vi "DataViewerMain_20190214.vi"() -> ()   [LabVIEW 2018]
uses:
  DataViewerStatesEnum.ctl
  HDF5/HDF5_NoiseInfoClust.ctl
  HDF5/TC_Data_Structure.ctl
  HDF5/HDF5_TC_Errors.ctl
  HDF5/AI_alarm_data_cluster.ctl
  <vilib>/addons/h5labview2/file/H5Fmode.ctl
  ItemsInFile_Clust.ctl
  <vilib>/addons/h5labview2/file/H5F.lvlib
  <vilib>/addons/h5labview2/group/H5G.lvlib
panel:
  in  "File Selection":string[](tree)
  out "Item Value":dbl[][](graph) caption="Beac_MaxValue"
  in  "1 Hz?":bool
  out "TimeStamp":dbl[](array[numeric])
  out "TimeString (High)":string[](array[string])
  in  "ReLoad Data":bool
  in  "Index#":cluster{dbl, dbl}(slide)={0.0, 2963.282178217822} scale=0.0..23219.0
  out "Current Time":timestamp
  in  "Exit":bool
  in  "Load Data":bool
  in  "Start Crawl":bool
  out "TimeString (Low)":string[](array[string])
  in  "Channel Selection":string[](tree)
  in  "path":path=path "C:/ConnexData"
  # "Ver 2019_05_28"
  # "Select a folder\n(Not an individual file)"
  # "Click Start Folder Crawl"
  # "Select a group, then \ndata set, then one or more\ndata files."
  # "Select whether the data is\non a 1 second or\n1 minute time scale"
  # "Click Load Selected Data"
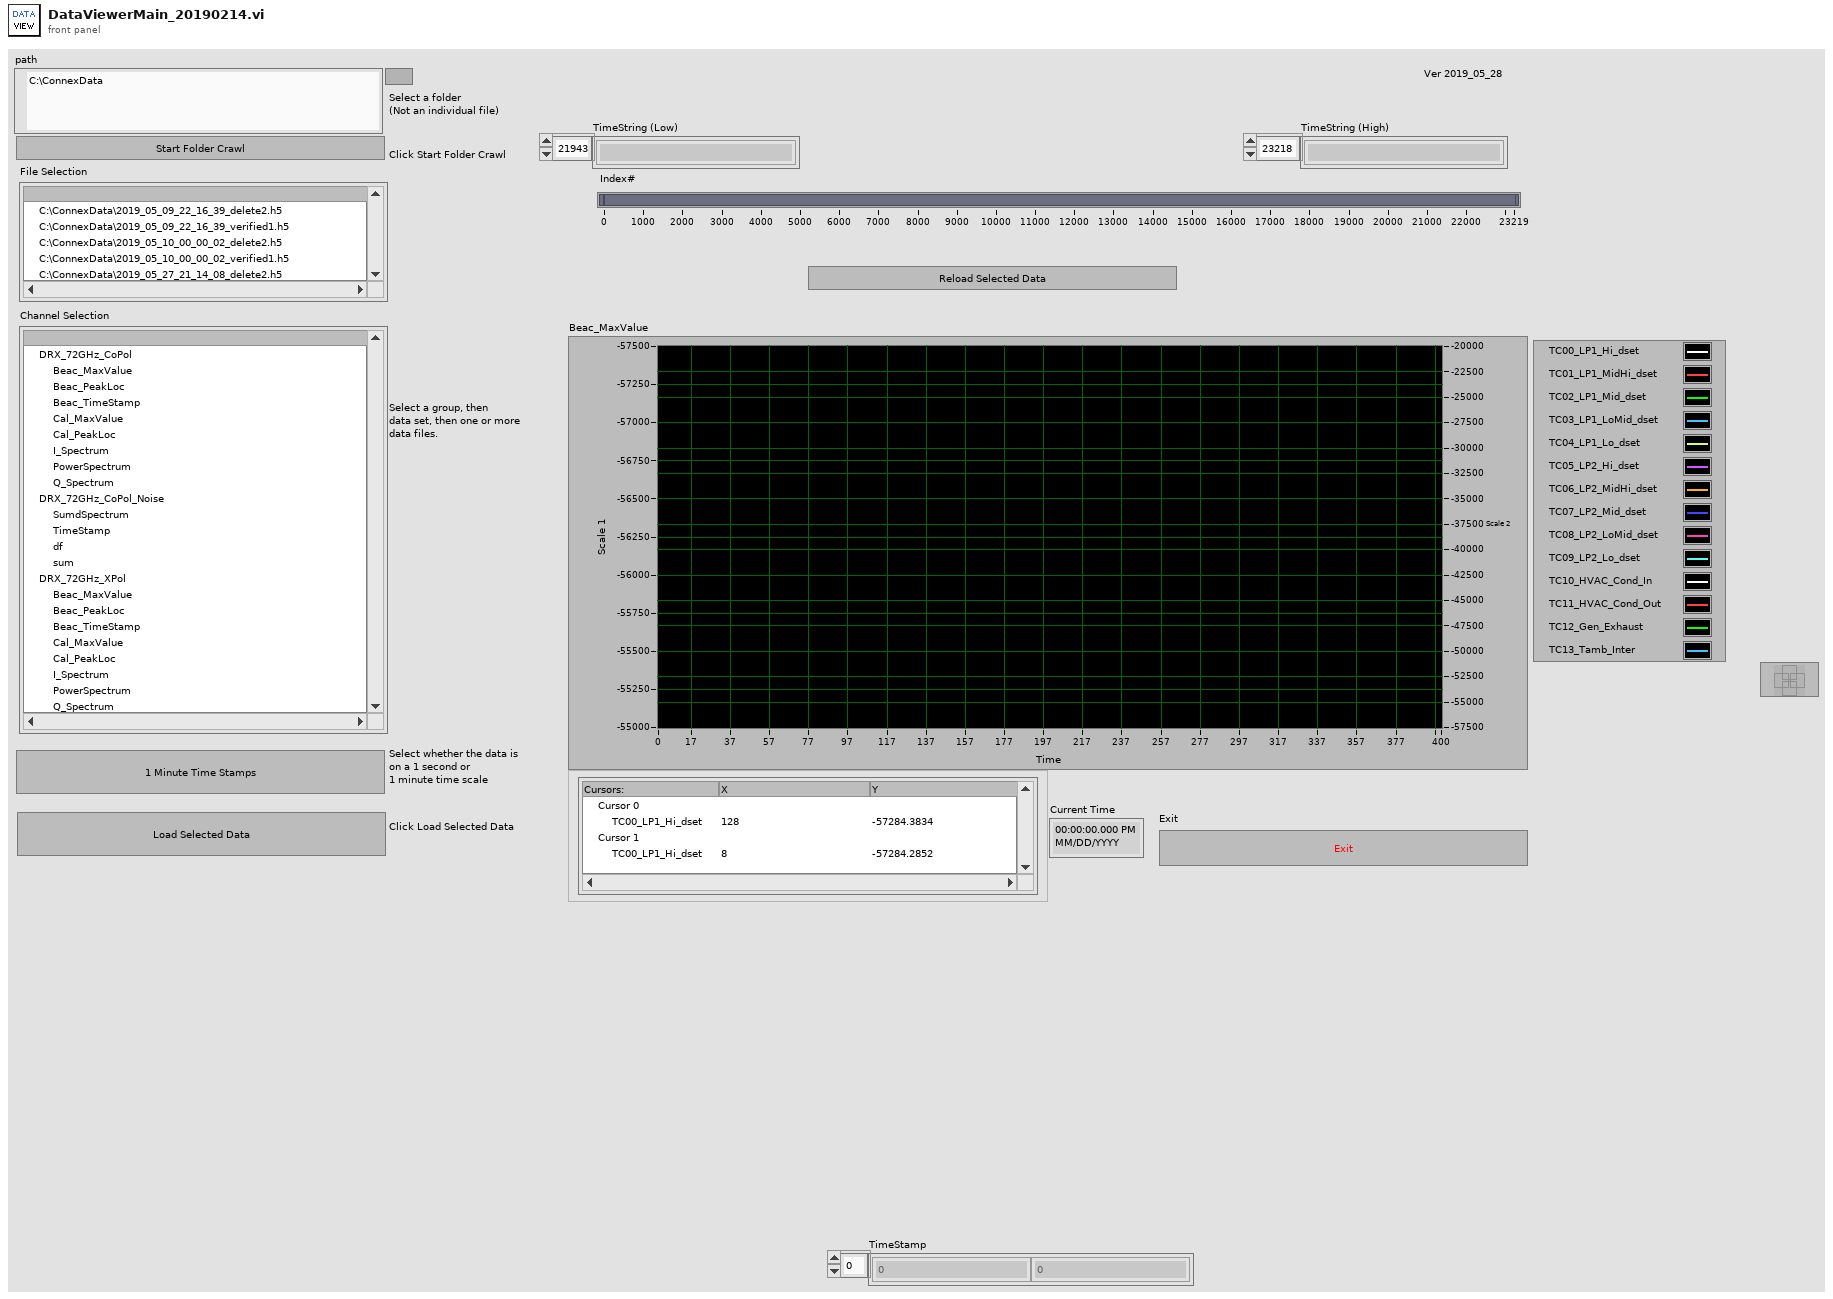
[diagram p1: front panel]
types:
  T1 = typedef "DataViewerStatesEnum.ctl" = enum16{"Idle", "Init", "CrawlFolders", "ListAllObjects", "PopulateTree", "LoadItemValues", "LoadBeacCalZoom", "LoadAlarms", "TimeShift", "Exit"}
  T2 = typedef "AI_alarm_data_cluster.ctl" = cluster{"current time":dbl, "date/time string":string, "AI 0":dbl, "AI 1":dbl, "AI 2":dbl, "AI 3":dbl, "AI 4":dbl, "AI 5":dbl, "AI 6":dbl, "AI 7":dbl, "AI 16":dbl, "AI 17":dbl, "AI 18":dbl, "AI 19":dbl, "AI 20":dbl, "AI 21":dbl, "AI 22":dbl, "AI 23":dbl}
  T3 = typedef "HDF5_TC_Errors.ctl" = cluster{"current time":dbl, "date/time string":string, "TC 0":dbl, "TC 1":dbl, "TC 2":dbl, "TC 3":dbl, "TC 4":dbl, "TC 5":dbl, "TC 6":dbl, "TC 7":dbl, "TC 8":dbl, "TC 9":dbl, "TC 10":dbl, "TC 11":dbl, "TC 12":dbl, "TC 13":dbl, "TC 14":dbl, "TC 15":dbl, "TC 16":dbl, "TC 17":dbl, "TC 18":dbl, "TC 19":dbl, "TC 20":dbl}
  T4 = typedef "TC_Data_Structure.ctl" = cluster{"TimeStamp":dbl, "TimeString":string, "TC0_LP1_Hi":dbl, "TC1_LP1_MidHi":dbl, "TC2_LP1_Mid":dbl, "TC3_LP1_LoMid":dbl, "TC4_LP1_Lo":dbl, "TC5_LP2_Hi":dbl, "TC6_LP2_MidHi":dbl, "TC7_LP2_Mid":dbl, "TC8_LP2_LoMid":dbl, "TC9_LP2_Lo":dbl, "TC10_HVAC_Cond_In":dbl, "TC11_HVAC_Cond_Out":dbl, "TC12_Gen_Exhaust":dbl, "TC13_Unused":dbl, "TC14_Unused":dbl, "TC15_Unused":dbl, "TC16_Unused":dbl, "TC17_Unused":dbl, "TC18_Unused":dbl, "TC19_Unused":dbl, "TC20_Unused":dbl, "TC21_Unused":dbl, "TC22_Unused":dbl, "TC23_Unused":dbl, "TC24_Unused":dbl, "TC25_Unused":dbl, "TC26_Unused":dbl, "TC27_Unused":dbl, "TC28_Unused":dbl, "TC29_Unused":dbl, "TC30_Unused":dbl, "TC31_Unused":dbl}
  T5 = typedef "HDF5_NoiseInfoClust.ctl" = cluster{"Timestring":string, "Timestamp":dbl, "df":dbl, "Sum":dbl}
  T6 = typedef "ItemsInFile_Clust.ctl" = cluster{"Group":string[], "Channel":string[][], "FilePath":string[]}
  T7 = typedef "H5F.lvlib/H5Fmode.ctl" = enum16{"read-only", "read-write", "overwrite", "create new", "open or create"}
  T8 = typedef "hid_t.ctl" = i32
  T9 = typedef "h5o_type.ctl" = enum8{"Group", "Dataset", "Named type"}
  T10 = cluster{"Left Cell String":string, "Child Text":string[], "Child Tag":string, "Item Indent":i32, "Child Only?":bool, "Glyph Index":i32}[]
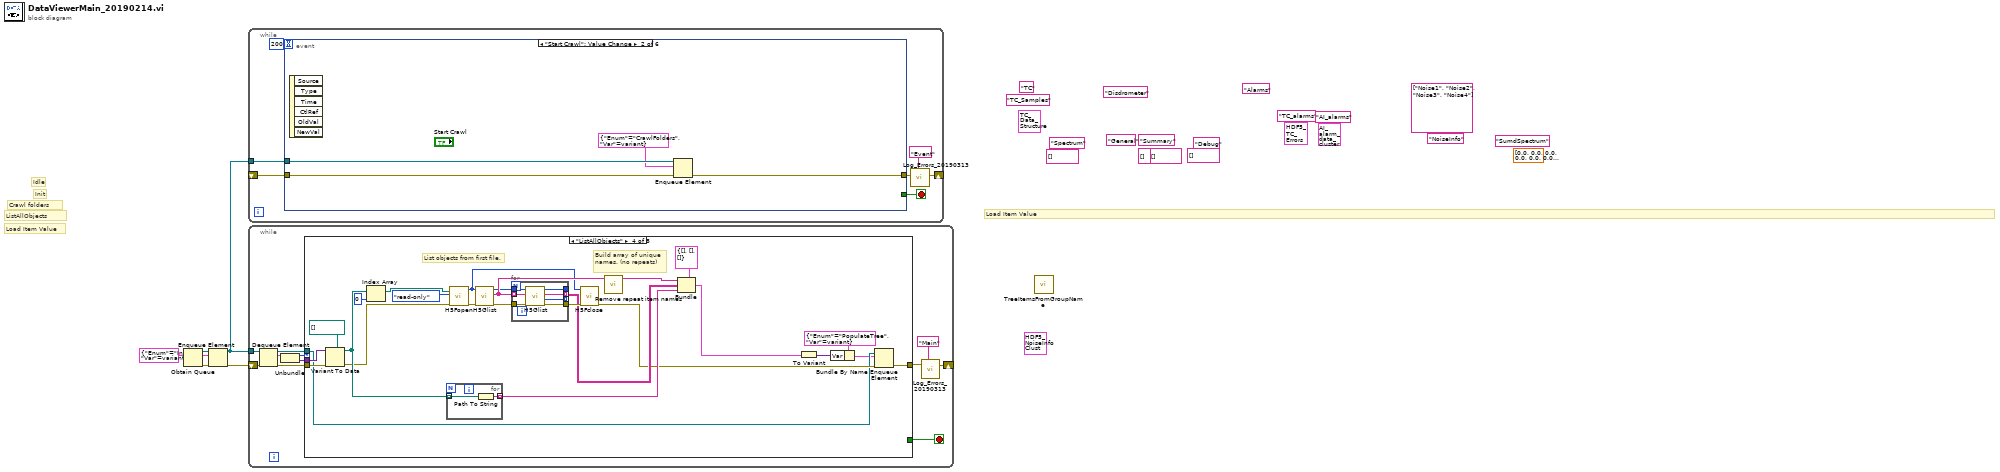
[diagram p0: block diagram]
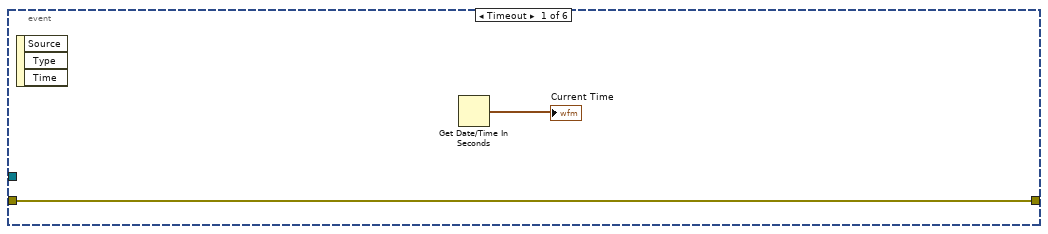
[diagram p2: hidden frame]
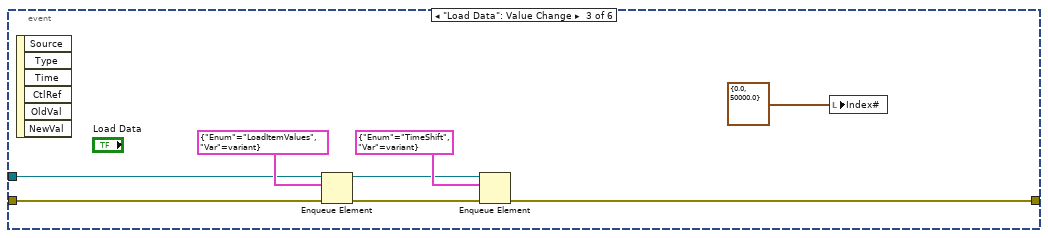
[diagram p3: hidden frame]
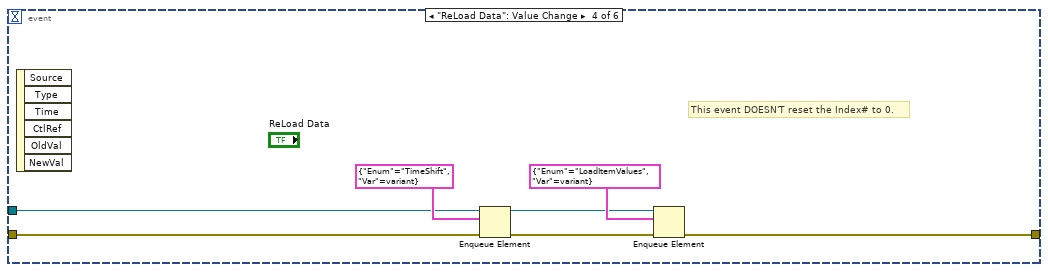
[diagram p4: hidden frame]
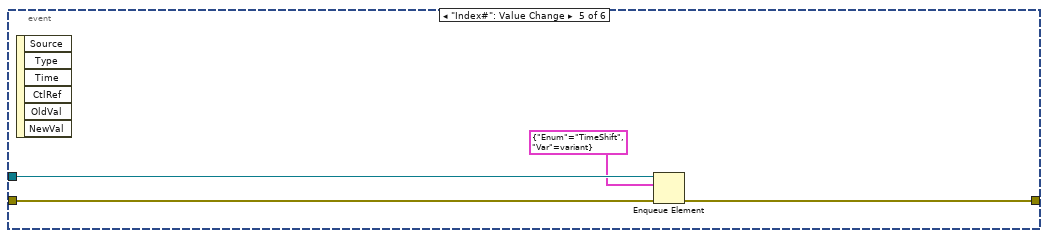
[diagram p5: hidden frame]
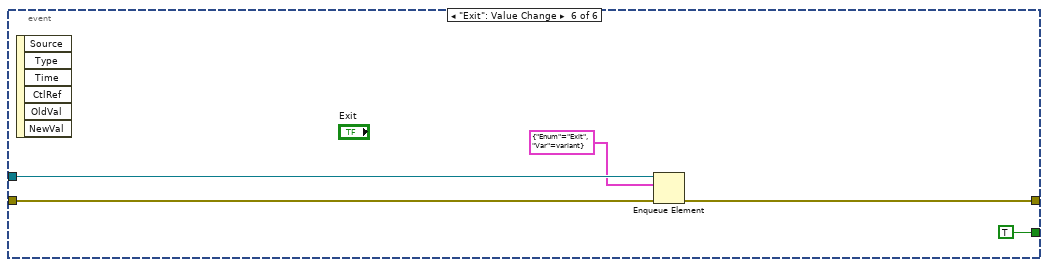
[diagram p6: hidden frame]
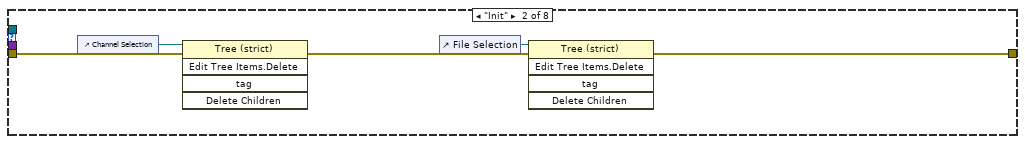
[diagram p8: hidden frame]
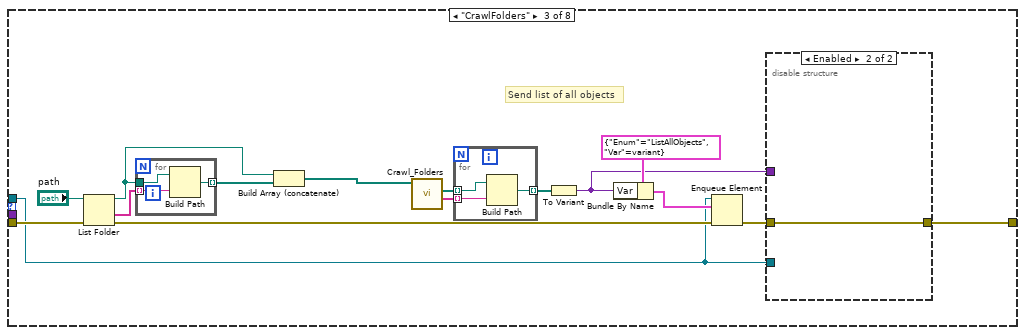
[diagram p9: hidden frame]
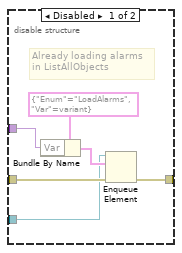
[diagram p10: hidden frame]
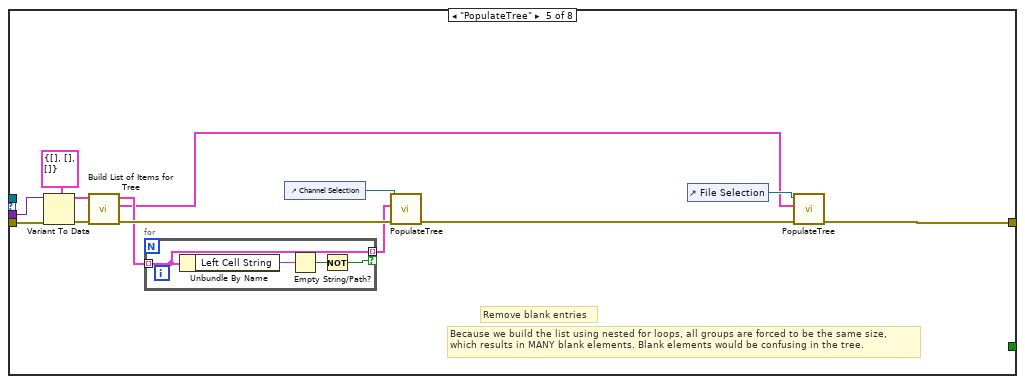
[diagram p11: hidden frame]
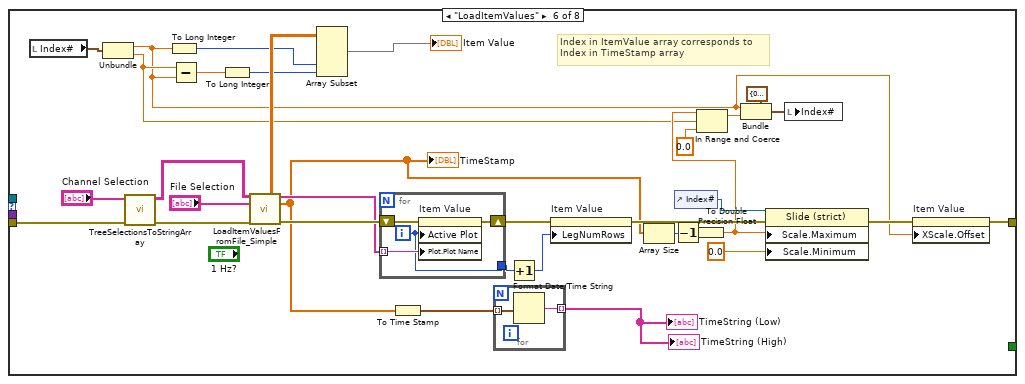
[diagram p12: hidden frame]
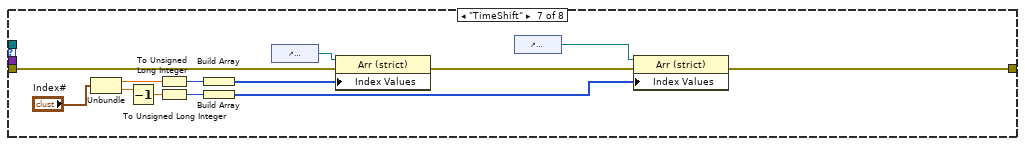
[diagram p13: hidden frame]
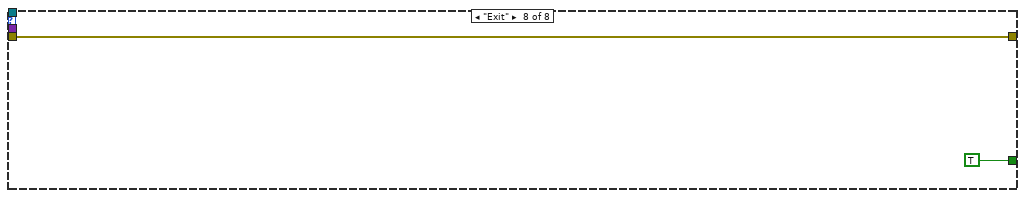
[diagram p14: hidden frame]
diagram:
  w2 = cluster{"Enum":T1, "Var":variant} {"Enum"=enum."Init", "Var"=variant}
  (unwired) string[] [] ("Debug Data")
  (unwired) string[] [] ("Debug Data")
  (unwired) string[] [] ("Spectrum Data")
  (unwired) string[] [] ("General Data")
  (unwired) dbl[] [0.0, 0.0, 0.0, 0.0, 0.0, 0.0, 0.0, 0.0, 0.0, 0.0, 0.0, 0.0, 0.0, 0.0, 0.0, 0.0, 0.0, 0.0, 0.0, 0.0, 0.0, 0.0, 0.0, 0.0, 0.0, 0.0, 0.0, 0.0, 0.0, 0.0, 0.0, 0.0, 0.0, 0.0, 0.0, 0.0, 0.0, 0.0, 0.0, 0.0, 0.0, 0.0, 0.0, 0.0, 0.0, 0.0, 0.0, 0.0, 0.0, 0.0, 0.0, 0.0, 0.0, 0.0, 0.0, 0.0, 0.0, 0.0, 0.0, 0.0, 0.0, 0.0, 0.0, 0.0, 0.0, 0.0, 0.0, 0.0, 0.0, 0.0, 0.0, 0.0, 0.0, 0.0, 0.0, 0.0, 0.0, 0.0, 0.0, 0.0, 0.0, 0.0, 0.0, 0.0, 0.0, 0.0, 0.0, 0.0, 0.0, 0.0, 0.0, 0.0, 0.0, 0.0, 0.0, 0.0, 0.0, 0.0, 0.0, 0.0, 0.0, 0.0, 0.0, 0.0, 0.0, 0.0, 0.0, 0.0, 0.0, 0.0, 0.0, 0.0, 0.0, 0.0, 0.0, 0.0, 0.0, 0.0, 0.0, 0.0, 0.0, 0.0, 0.0, 0.0, 0.0, 0.0, 0.0, 0.0, 0.0, 0.0, 0.0, 0.0, 0.0, 0.0, 0.0, 0.0, 0.0, 0.0, 0.0, 0.0, 0.0, 0.0, 0.0, 0.0, 0.0, 0.0, 0.0, 0.0, 0.0, 0.0, 0.0, 0.0, 0.0, 0.0, 0.0, 0.0, 0.0, 0.0, 0.0, 0.0, 0.0, 0.0, 0.0, 0.0, 0.0, 0.0, 0.0, 0.0, 0.0, 0.0, 0.0, 0.0, 0.0, 0.0, 0.0, 0.0, 0.0, 0.0, 0.0, 0.0, 0.0, 0.0, 0.0, 0.0, 0.0, 0.0, 0.0, 0.0, 0.0, 0.0, 0.0, 0.0, 0.0, 0.0, 0.0, 0.0, 0.0, 0.0, 0.0, 0.0, 0.0, 0.0, 0.0, 0.0, 0.0, 0.0, 0.0, 0.0, 0.0, 0.0, 0.0, 0.0, 0.0, 0.0, 0.0, 0.0, 0.0, 0.0, 0.0, 0.0, 0.0, 0.0, 0.0, 0.0, 0.0, 0.0, 0.0, 0.0, 0.0, 0.0, 0.0, 0.0, 0.0, 0.0, 0.0, 0.0, 0.0, 0.0, 0.0, 0.0, 0.0, 0.0, 0.0, 0.0, 0.0, 0.0, 0.0, 0.0, 0.0, 0.0, 0.0, 0.0, 0.0, 0.0, 0.0, 0.0, 0.0, 0.0, 0.0, 0.0, 0.0, 0.0, 0.0, 0.0, 0.0, 0.0, 0.0, 0.0, 0.0, 0.0, 0.0, 0.0, 0.0, 0.0, 0.0, 0.0, 0.0, 0.0, 0.0, 0.0, 0.0, 0.0, 0.0, 0.0, 0.0, 0.0, 0.0, 0.0, 0.0, 0.0, 0.0, 0.0, 0.0, 0.0, 0.0, 0.0, 0.0, 0.0, 0.0, 0.0, 0.0, 0.0, 0.0, 0.0, 0.0, 0.0, 0.0, 0.0, 0.0, 0.0, 0.0, 0.0, 0.0, 0.0, 0.0, 0.0, 0.0, 0.0, 0.0, 0.0, 0.0, 0.0, 0.0, 0.0, 0.0, 0.0, 0.0, 0.0, 0.0, 0.0, 0.0, 0.0, 0.0, 0.0, 0.0, 0.0, 0.0, 0.0, 0.0, 0.0, 0.0, 0.0, 0.0, 0.0, 0.0, 0.0, 0.0, 0.0, 0.0, 0.0, 0.0, 0.0, 0.0, 0.0, 0.0, 0.0, 0.0, 0.0, 0.0, 0.0, 0.0, 0.0, 0.0, 0.0, 0.0, 0.0, 0.0, 0.0, 0.0, 0.0, 0.0, 0.0, 0.0, 0.0, 0.0, 0.0, 0.0, 0.0, 0.0, 0.0, 0.0, 0.0, 0.0, 0.0, 0.0, 0.0, 0.0, 0.0, 0.0, 0.0, 0.0, 0.0, 0.0, 0.0, 0.0, 0.0, 0.0, 0.0, 0.0, 0.0, 0.0, 0.0, 0.0, 0.0, 0.0, 0.0, 0.0, 0.0, 0.0, 0.0, 0.0, 0.0, 0.0, 0.0, 0.0, 0.0, 0.0, 0.0, 0.0, 0.0, 0.0, 0.0, 0.0, 0.0, 0.0, 0.0, 0.0, 0.0, 0.0, 0.0, 0.0, 0.0, 0.0, 0.0, 0.0, 0.0, 0.0, 0.0, 0.0, 0.0, 0.0, 0.0, 0.0, 0.0, 0.0, 0.0, 0.0, 0.0, 0.0, 0.0, 0.0, 0.0, 0.0, 0.0, 0.0, 0.0, 0.0, 0.0, 0.0, 0.0, 0.0, 0.0, 0.0, 0.0, 0.0, 0.0, 0.0, 0.0, 0.0, 0.0, 0.0, 0.0, 0.0, 0.0, 0.0, 0.0, 0.0, 0.0, 0.0, 0.0, 0.0, 0.0, 0.0, 0.0, 0.0, 0.0, 0.0, 0.0, 0.0, 0.0, 0.0, 0.0, 0.0, 0.0, 0.0, 0.0, 0.0, 0.0, 0.0, 0.0, 0.0, 0.0, 0.0, 0.0, 0.0, 0.0, 0.0, 0.0, 0.0, 0.0, 0.0, 0.0, 0.0, 0.0, 0.0, 0.0, 0.0, 0.0, 0.0, 0.0, 0.0, 0.0, 0.0, 0.0, 0.0, 0.0, 0.0, 0.0, 0.0, 0.0, 0.0, 0.0, 0.0, 0.0, 0.0, 0.0, 0.0, 0.0, 0.0, 0.0, 0.0, 0.0, 0.0, 0.0, 0.0, 0.0, 0.0, 0.0, 0.0, 0.0, 0.0, 0.0, 0.0, 0.0, 0.0, 0.0, 0.0, 0.0, 0.0, 0.0, 0.0, 0.0, 0.0, 0.0, 0.0, 0.0, 0.0, 0.0, 0.0, 0.0, 0.0, 0.0, 0.0, 0.0, 0.0, 0.0, 0.0, 0.0, 0.0, 0.0, 0.0, 0.0, 0.0, 0.0, 0.0, 0.0, 0.0, 0.0, 0.0, 0.0, 0.0, 0.0, 0.0, 0.0, 0.0, 0.0, 0.0, 0.0, 0.0, 0.0, 0.0, 0.0, 0.0, 0.0, 0.0, 0.0, 0.0, 0.0, 0.0, 0.0, 0.0, 0.0, 0.0, 0.0, 0.0, 0.0, 0.0, 0.0, 0.0, 0.0, 0.0, 0.0, 0.0, 0.0, 0.0, 0.0, 0.0, 0.0, 0.0, 0.0, 0.0, 0.0, 0.0, 0.0, 0.0, 0.0, 0.0, 0.0, 0.0, 0.0, 0.0, 0.0, 0.0, 0.0, 0.0, 0.0, 0.0, 0.0, 0.0, 0.0, 0.0, 0.0, 0.0, 0.0, 0.0, 0.0, 0.0, 0.0, 0.0, 0.0, 0.0, 0.0, 0.0, 0.0, 0.0, 0.0, 0.0, 0.0, 0.0, 0.0, 0.0, 0.0, 0.0, 0.0, 0.0, 0.0, 0.0, 0.0, 0.0, 0.0, 0.0, 0.0, 0.0, 0.0, 0.0, 0.0, 0.0, 0.0, 0.0, 0.0, 0.0, 0.0, 0.0, 0.0, 0.0, 0.0, 0.0, 0.0, 0.0, 0.0, 0.0, 0.0, 0.0, 0.0, 0.0, 0.0, 0.0, 0.0, 0.0, 0.0, 0.0, 0.0, 0.0, 0.0, 0.0, 0.0, 0.0, 0.0, 0.0, 0.0, 0.0, 0.0, 0.0, 0.0, 0.0, 0.0, 0.0, 0.0, 0.0, 0.0, 0.0, 0.0, 0.0, 0.0, 0.0, 0.0, 0.0, 0.0, 0.0, 0.0, 0.0, 0.0, 0.0, 0.0, 0.0, 0.0, 0.0, 0.0, 0.0, 0.0, 0.0, 0.0, 0.0, 0.0, 0.0, 0.0, 0.0, 0.0, 0.0, 0.0, 0.0, 0.0, 0.0, 0.0, 0.0, 0.0, 0.0, 0.0, 0.0, 0.0, 0.0, 0.0, 0.0, 0.0, 0.0, 0.0, 0.0, 0.0, 0.0, 0.0, 0.0, 0.0, 0.0, 0.0, 0.0, 0.0, 0.0, 0.0, 0.0, 0.0, 0.0, 0.0, 0.0, 0.0, 0.0, 0.0, 0.0, 0.0, 0.0, 0.0, 0.0, 0.0, 0.0, 0.0, 0.0, 0.0, 0.0, 0.0, 0.0, 0.0, 0.0, 0.0, 0.0, 0.0, 0.0, 0.0, 0.0, 0.0, 0.0, 0.0, 0.0, 0.0, 0.0, 0.0, 0.0, 0.0, 0.0, 0.0, 0.0, 0.0, 0.0, 0.0, 0.0, 0.0, 0.0, 0.0, 0.0, 0.0, 0.0, 0.0, 0.0, 0.0, 0.0, 0.0, 0.0, 0.0, 0.0, 0.0, 0.0, 0.0, 0.0, 0.0, 0.0, 0.0, 0.0, 0.0, 0.0, 0.0, 0.0, 0.0, 0.0, 0.0, 0.0, 0.0, 0.0, 0.0, 0.0, 0.0, 0.0, 0.0, 0.0, 0.0, 0.0, 0.0, 0.0, 0.0, 0.0, 0.0, 0.0, 0.0, 0.0, 0.0, 0.0, 0.0, 0.0, 0.0, 0.0, 0.0, 0.0, 0.0, 0.0, 0.0, 0.0, 0.0, 0.0, 0.0, 0.0, 0.0, 0.0, 0.0, 0.0, 0.0, 0.0, 0.0, 0.0, 0.0, 0.0, 0.0, 0.0, 0.0, 0.0, 0.0, 0.0, 0.0, 0.0, 0.0, 0.0, 0.0, 0.0, 0.0, 0.0, 0.0, 0.0, 0.0, 0.0, 0.0, 0.0, 0.0, 0.0, 0.0, 0.0, 0.0, 0.0, 0.0, 0.0, 0.0, 0.0, 0.0, 0.0, 0.0, 0.0, 0.0, 0.0, 0.0, 0.0, 0.0, 0.0, 0.0, 0.0, 0.0, 0.0, 0.0, 0.0, 0.0, 0.0, 0.0, 0.0, 0.0, 0.0, 0.0, 0.0, 0.0, 0.0, 0.0, 0.0, 0.0, 0.0, 0.0, 0.0, 0.0, 0.0, 0.0, 0.0, 0.0, 0.0, 0.0, 0.0, 0.0, 0.0, 0.0, 0.0, 0.0, 0.0, 0.0, 0.0, 0.0, 0.0, 0.0, 0.0, 0.0, 0.0, 0.0, 0.0, 0.0, 0.0, 0.0, 0.0, 0.0, 0.0, 0.0, 0.0, 0.0, 0.0, 0.0, 0.0, 0.0, 0.0, 0.0, 0.0, 0.0, 0.0, 0.0, 0.0, 0.0, 0.0, 0.0, 0.0, 0.0, 0.0, 0.0, 0.0, 0.0, 0.0, 0.0] ("SumdSpectrum")
  (unwired) T2 {"current time"=0.0, "date/time string"="", "AI 0"=0.0, "AI 1"=0.0, "AI 2"=0.0, "AI 3"=0.0, "AI 4"=0.0, "AI 5"=0.0, "AI 6"=0.0, "AI 7"=0.0, "AI 16"=0.0, "AI 17"=0.0, "AI 18"=0.0, "AI 19"=0.0, "AI 20"=0.0, "AI 21"=0.0, "AI 22"=0.0, "AI 23"=0.0} ("AI_alarm_Clust")
  (unwired) T3 {"current time"=0.0, "date/time string"="", "TC 0"=0.0, "TC 1"=0.0, "TC 2"=0.0, "TC 3"=0.0, "TC 4"=0.0, "TC 5"=0.0, "TC 6"=0.0, "TC 7"=0.0, "TC 8"=0.0, "TC 9"=0.0, "TC 10"=0.0, "TC 11"=0.0, "TC 12"=0.0, "TC 13"=0.0, "TC 14"=0.0, "TC 15"=0.0, "TC 16"=0.0, "TC 17"=0.0, "TC 18"=0.0, "TC 19"=0.0, "TC 20"=0.0} ("TC_alarm")
  (unwired) "SumdSpectrum" ("string")
  (unwired) "NoiseInfo" ("string")
  (unwired) "TC" ("name")
  (unwired) T4 {"TimeStamp"=0.0, "TimeString"="", "TC0_LP1_Hi"=0.0, "TC1_LP1_MidHi"=0.0, "TC2_LP1_Mid"=0.0, "TC3_LP1_LoMid"=0.0, "TC4_LP1_Lo"=0.0, "TC5_LP2_Hi"=0.0, "TC6_LP2_MidHi"=0.0, "TC7_LP2_Mid"=0.0, "TC8_LP2_LoMid"=0.0, "TC9_LP2_Lo"=0.0, "TC10_HVAC_Cond_In"=0.0, "TC11_HVAC_Cond_Out"=0.0, "TC12_Gen_Exhaust"=0.0, "TC13_Unused"=0.0, "TC14_Unused"=0.0, "TC15_Unused"=0.0, "TC16_Unused"=0.0, "TC17_Unused"=0.0, "TC18_Unused"=0.0, "TC19_Unused"=0.0, "TC20_Unused"=0.0, "TC21_Unused"=0.0, "TC22_Unused"=0.0, "TC23_Unused"=0.0, "TC24_Unused"=0.0, "TC25_Unused"=0.0, "TC26_Unused"=0.0, "TC27_Unused"=0.0, "TC28_Unused"=0.0, "TC29_Unused"=0.0, "TC30_Unused"=0.0, "TC31_Unused"=0.0} ("HDF5_TCInfo")
  (unwired) "General" ("string")
  (unwired) "Spectrum" ("string")
  (unwired) "Debug" ("string")
  (unwired) "Summary" ("string")
  (unwired) "Disdrometer" ("name")
  (unwired) "Alarms" ("name")
  (unwired) "AI_alarms" ("string")
  (unwired) "TC_alarms" ("string")
  (unwired) string[] ["Noise1", "Noise2", "Noise3", "Noise4"]
  (unwired) "TC_Samples" ("string")
  (unwired) T5 {"Timestring"="Timestamp string goes here", "Timestamp"=0.0, "df"=7629.39453125, "Sum"=0.0} ("HDF5_NoiseInfo")
  # "Load Item Value"
  # "ListAllObjects"
  # "Crawl folders"
  # "Init"
  # "Idle"
  # "Load Item Value"
  n1 = Obtain Queue(element data type=w2) -> (queue out=w5:refnum<queue>, error out=w4:errorcluster)  [unwired: 4 in, 1 out]
  n2 = Enqueue Element(queue=w5, element=w2, error in (no error)=w4) -> (queue out=w1:refnum<queue>, error out=w3:errorcluster)  [unwired: 1 in, 1 out]
  n3 = while {
    shift-right: [w11] -> _
    shift-left: _ -> [w9]
    tunnel: w1 -> [w8]
    stop <- w7 stop-if-true
    n4 = event shown="[1] \"Start Crawl\": Value Change" {
      selector: _ -> [_ _ _ _ _ _]
      dyn-events: _ -> [_ _ _ _ _ _]
      timeout: 200 -> [_ _ _ _ _ _]
      tunnel: [w14 w18 w21 w32 w36 w41] -> w12
      tunnel: w9 -> [w14 w17 w23 w31 w35 w40]
      tunnel: w8 -> [_ w16 w20 w27 w34 w39]
      tunnel: [_ _ _ _ _ TRUE] -> w7
      event Timeout {
        n5 = event-data() -> ()  [unwired: 1 in, 3 out]
        n6 = Get Date/Time In Seconds() -> (seconds since 1Jan1904=→"Current Time":timestamp)
      }
      event "Start Crawl": Value Change {
        n7 = event-data() -> ()  [unwired: 1 in, 6 out]
        n8 = Enqueue Element(queue=w16, element=cluster{"Enum":T1, "Var":variant} {"Enum"=enum."CrawlFolders", "Var"=variant}, error in (no error)=w17) -> (error out=w18:errorcluster)  [unwired: 1 in, 2 out]
      }
      event "Load Data": Value Change {
        n9 = event-data() -> ()  [unwired: 1 in, 6 out]
        n10 = Enqueue Element(queue=w20, element=cluster{"Enum":T1, "Var":variant} {"Enum"=enum."LoadItemValues", "Var"=variant}, error in (no error)=w23) -> (queue out=w19:refnum<queue>, error out=w22:errorcluster)  [unwired: 1 in, 1 out]
        n11 = Enqueue Element(queue=w19, element=cluster{"Enum":T1, "Var":variant} {"Enum"=enum."TimeShift", "Var"=variant}, error in (no error)=w22) -> (error out=w21:errorcluster)  [unwired: 1 in, 2 out]
        n12 = local write "Index#"(cluster{dbl, dbl} {0.0, 50000.0} ("Index#")) -> ()
      }
      event "ReLoad Data": Value Change {
        # "This event DOESN'T reset the Index# to 0."
        n13 = event-data() -> ()  [unwired: 1 in, 6 out]
        n14 = Enqueue Element(queue=w27, element=cluster{"Enum":T1, "Var":variant} {"Enum"=enum."TimeShift", "Var"=variant}) -> (queue out=w28:refnum<queue>)  [unwired: 2 in, 2 out]
        n15 = Enqueue Element(queue=w28, element=cluster{"Enum":T1, "Var":variant} {"Enum"=enum."LoadItemValues", "Var"=variant}, error in (no error)=w31) -> (error out=w32:errorcluster)  [unwired: 1 in, 2 out]
      }
      event "Index#": Value Change {
        n16 = event-data() -> ()  [unwired: 1 in, 6 out]
        n17 = Enqueue Element(queue=w34, element=cluster{"Enum":T1, "Var":variant} {"Enum"=enum."TimeShift", "Var"=variant}, error in (no error)=w35) -> (error out=w36:errorcluster)  [unwired: 1 in, 2 out]
      }
      event "Exit": Value Change {
        n18 = event-data() -> ()  [unwired: 1 in, 6 out]
        n19 = Enqueue Element(queue=w39, element=cluster{"Enum":T1, "Var":variant} {"Enum"=enum."Exit", "Var"=variant}, error in (no error)=w40) -> (error out=w41:errorcluster)  [unwired: 1 in, 2 out]
      }
    }
    n20 = call "Log_Errors_20190313.vi"("LoopName"="Event", "error in"=w12) -> ("error out"=w11:errorcluster)  [unwired: 9 in]
  }
  n21 = while {
    tunnel: w1 -> [w42]
    shift-right: [w47] -> _
    shift-left: w3 -> [w52]
    stop <- w44 stop-if-true
    n22 = Dequeue Element(queue=w42, error in (no error)=w52) -> (queue out=w45:refnum<queue>, element=w51:cluster{"Enum":T1, "Var":variant}, error out=w49:errorcluster)  [unwired: 1 in, 1 out]
    n23 = Unbundle(w51) -> ("Enum"=w50:T1, "Var"=w46:variant)
    n24 = case shown="\"ListAllObjects\"" w50 {
      tunnel: w49 -> [w53 w57 w69 w112 w134 w169 w187 w190]
      tunnel: [w53 w55 w61 w98 w124 w140 w186 w190] -> w48
      tunnel: w46 -> [_ _ _ w111 w133 _ _ _]
      tunnel: w45 -> [_ _ w60 w94 _ _ _ _]
      tunnel: [_ _ _ _ _ _ _ TRUE] -> w44
      frame "Idle", Default {
        # "We might not use this case.\nLuke 2-21-2018"
      }
      frame "Init" {
        n25 = control-ref of="Channel Selection"() -> (w58:refnum<vi>)
        n26 = invoke on="Invoke Node" class="Tree (strict)" method="Edit Tree Items.Delete"(reference=w58, error in=w57) -> (error out=w56:errorcluster)  [unwired: 3 in, 4 out]
        n27 = control-ref of="File Selection"() -> (w54:refnum<vi>)
        n28 = invoke on="Invoke Node" class="Tree (strict)" method="Edit Tree Items.Delete"(reference=w54, error in=w56) -> (error out=w55:errorcluster)  [unwired: 3 in, 4 out]
      }
      frame "CrawlFolders" {
        # "Send list of all objects"
        n29 = List Folder(path="path", error in=w69) -> (path out=w63:path, folder names=w71:string[], error out=w65:errorcluster)  [unwired: 2 in, 1 out]
        n30 = for {
          tunnel: w71 -> [w87] mode=indexing
          tunnel: w63 -> [w86]
          tunnel: [w85] -> w72 mode=indexing
          n31 = Build Path(base path=w86, name or relative path=w87) -> (appended path=w85:path)
        }
        n32 = Build Array (concatenate)(w63, w72) -> (w64:path[])
        n33 = call "Crawl_Folders.vi"("path in"=w64) -> ("FileNames"=w74:string[], "Folders"=w73:path[])  [unwired: 9 in]
        n34 = for {
          tunnel: w74 -> [w83] mode=indexing
          tunnel: w73 -> [w84] mode=indexing
          tunnel: [w82] -> w66 mode=indexing
          n35 = Build Path(base path=w84, name or relative path=w83) -> (appended path=w82:path)
        }
        n36 = To Variant(anything=w66) -> (Variant=w59:variant)
        n37 = Bundle By Name(cluster=cluster{"Enum":T1, "Var":variant} {"Enum"=enum."ListAllObjects", "Var"=variant}, "Var"=w59) -> (w67:cluster{"Enum":T1, "Var":variant})
        n38 = Enqueue Element(queue=w60, element=w67, error in (no error)=w65) -> (error out=w62:errorcluster)  [unwired: 1 in, 2 out]
        n39 = disable-structure shown="Enabled" {
          disable-tunnel: w62 -> [w78 w81]
          disable-tunnel: [w77 w81] -> w61
          disable-tunnel: w60 -> [w76 _]
          disable-tunnel: w59 -> [w75 _]
          frame Disabled {
            # "Already loading alarms\nin ListAllObjects"
            n40 = Bundle By Name(cluster=cluster{"Enum":T1, "Var":variant} {"Enum"=enum."LoadAlarms", "Var"=variant}, "Var"=w75) -> (w80:cluster{"Enum":T1, "Var":variant})
            n41 = Enqueue Element(queue=w76, element=w80, error in (no error)=w78) -> (error out=w77:errorcluster)  [unwired: 1 in, 2 out]
          }
          frame Enabled {
          }
        }
      }
      frame "ListAllObjects" {
        # "List objects from first file."
        # "Build array of unique names. (no repeats)"
        n42 = Variant To Data(error in=w112, type=path[] [], Variant=w111) -> (data=w103:path[], error out=w102:errorcluster)
        n43 = Index Array(array=w103, index=0) -> (element=w108:path)
        n44 = for {
          tunnel: w103 -> [w121] mode=indexing
          tunnel: [w120] -> w99 mode=indexing
          n45 = Path To String(path=w121) -> (string=w120:string)
        }
        n46 = call <vilib>:"H5Fopen.vi"("error in (no error)"=w102, "mode (read-only)"=H5Fmode."read-only" ("mode"), "path"=w108) -> ("error out"=w105:errorcluster, "ref out"=w88:T8)  [unwired: 7 in]
        n47 = call <vilib>:"H5Glist.vi"("error in (no error)"=w105, "ref in"=w88) -> ("error out"=w106:errorcluster, "names"=w109:string[], "ref out"=w90:T8)  [unwired: 6 in, 1 out]
        n48 = for {
          tunnel: w90 -> [w119]
          tunnel: w109 -> [w118] mode=indexing
          tunnel: w106 -> [w117]
          tunnel: [w116] -> w107
          tunnel: [w115] -> _
          tunnel: [w114] -> w100 mode=indexing
          tunnel: [w113] -> _ mode=indexing
          n49 = call <vilib>:"H5Glist.vi"("error in (no error)"=w117, "group (.)"=w118, "ref in"=w119) -> ("error out"=w116:errorcluster, "types"=w113:T9[], "names"=w114:string[], "ref out"=w115:T8)  [unwired: 5 in]
        }
        n50 = call <vilib>:"H5Fclose.vi"("error in (no error)"=w107, "ref"=w88) -> ("error out"=w97:errorcluster)  [unwired: 9 in]
        n51 = call "Remove repeat item names.vi"("names"=w109) -> ("Array"=w101:string[])  [unwired: 10 in]
        n52 = Bundle(cluster=T6 {"Group"=[], "Channel"=[], "FilePath"=[]} ("output cluster"), "Group"=w101, "Channel"=w100, "FilePath"=w99) -> (w95:T6)
        n53 = To Variant(anything=w95) -> (Variant=w93:variant)
        n54 = Bundle By Name(cluster=cluster{"Enum":T1, "Var":variant} {"Enum"=enum."PopulateTree", "Var"=variant}, "Var"=w93) -> (w92:cluster{"Enum":T1, "Var":variant})
        n55 = Enqueue Element(queue=w94, element=w92, error in (no error)=w97) -> (error out=w98:errorcluster)  [unwired: 1 in, 2 out]
      }
      frame "PopulateTree" {
        # "Because we build the list using nested for loops, all groups are forced to be the same size,\nwhich results in MANY blank elements. Blank elements would be confusing in the tree."
        # "Remove blank entries"
        n56 = Variant To Data(error in=w134, type=T6 {"Group"=[], "Channel"=[], "FilePath"=[]} ("output cluster"), Variant=w133) -> (data=w131:T6, error out=w132:errorcluster)
        n57 = call "Build List of Items for Tree.vi"("error in (no error)"=w132, "output cluster"=w131) -> ("error out"=w128:errorcluster, "FileTree"=w122:T10, "TreeItems"=w127:T10)  [unwired: 7 in]
        n58 = for {
          tunnel: w127 -> [w137] mode=indexing
          tunnel: [w137] -> w126 mode=indexing if=w135
          n59 = Unbundle By Name(w137) -> ("Left Cell String"=w138:string)
          n60 = Empty String/Path?(string/path=w138) -> (empty?=w136:bool)
          n61 = Not(x=w136) -> (.not. x?=w135:bool)
        }
        n62 = control-ref of="Channel Selection"() -> (w129:refnum<vi>)
        n63 = call "PopulateTree.vi"("error in (no error)"=w128, "Array"=w126, "TreeControl in"=w129) -> ("error out"=w125:errorcluster)  [unwired: 8 in]
        n64 = control-ref of="File Selection"() -> (w123:refnum<vi>)
        n65 = call "PopulateTree.vi"("error in (no error)"=w125, "Array"=w122, "TreeControl in"=w123) -> ("error out"=w124:errorcluster)  [unwired: 8 in]
      }
      frame "LoadItemValues" {
        # "Index in ItemValue array corresponds to\nIndex in TimeStamp array"
        n66 = local read "Index#"() -> (w164:cluster{dbl, dbl})
        n67 = Unbundle(w164) -> (w139:dbl, w143:dbl)
        n68 = call "TreeSelectionsToStringArray.vi"("error in (no error)"=w169, "Channel Selection"="Channel Selection") -> ("error out"=w159:errorcluster, "Array"=w160:string[][])  [unwired: 8 in]
        n69 = To Long Integer(number=w139) -> (32bit integer=w152:i32)
        n70 = Subtract(x=w143, y=w139) -> (x-y=w163:dbl)
        n71 = To Long Integer(number=w163) -> (32bit integer=w151:i32)
        n72 = call "LoadItemValuesFromFile_Simple.vi"("Array in"=w160, "FileArray"="File Selection", "error in (no error)"=w159) -> ("Values"=w166:dbl[][], "Item"=w157:string[], "Time 60/min"=w149:dbl[], "error out"=w170:errorcluster)  [unwired: 9 in]
        "TimeStamp" <- w149
        n73 = Array Subset(array=w166, index (col)=w152, length (col)=w151) -> (→"Item Value":dbl[][])  [unwired: 2 in]
        n74 = for {
          tunnel: w157 -> [w173] mode=indexing
          shift-right: [w174] -> w156
          shift-left: w170 -> [w175]
          tunnel: [w172] -> w154
          i -> [w172]
          n75 = property on="Item Value" class="WFGraph (strict)"(error in=w175, "Active Plot"=w172, "Plot.Plot Name"=w173) -> (error out=w174:errorcluster)  [unwired: 1 in, 1 out]
        }
        n76 = To Time Stamp(1:w149) -> (0:w162:timestamp[])
        n77 = for {
          tunnel: w162 -> [w177] mode=indexing
          tunnel: [w176] -> w161 mode=indexing
          n78 = Format Date/Time String(seconds (now)=w177) -> (date/time string=w176:string)  [unwired: 2 in]
        }
        "TimeString (Low)" <- w161
        "TimeString (High)" <- w161
        n79 = Increment(x=w154) -> (x+1=w153:i32)
        n80 = property on="Item Value" class="WFGraph (strict)"(error in=w156, "LegNumRows"=w153) -> (error out=w155:errorcluster)  [unwired: 1 in, 1 out]
        n81 = Array Size(array=w149) -> (size(s)=w167:i32)
        n82 = Decrement(x=w167) -> (x-1=w150:i32)
        n83 = control-ref of="Index#"() -> (w168:refnum<vi>)
        n84 = To Double Precision Float(number=w150) -> (double precision float=w145:dbl)
        n85 = In Range and Coerce(upper limit=w145, x=w143, lower limit=0.0 ("x")) -> (coerced(x)=w142:dbl)  [unwired: 1 out]
        n86 = Bundle(cluster=cluster{dbl, dbl} {0.0, 50000.0} ("Index#"), w139, w142) -> (w147:cluster{dbl, dbl})
        n87 = property class="Slide (strict)"(reference=w168, error in=w155, "Scale.Maximum"=w145, "Scale.Minimum"=0.0 ("Scale.Range:Minimum")) -> (error out=w141:errorcluster)  [unwired: 1 out]
        n88 = local write "Index#"(w147) -> ()
        n89 = property on="Item Value" class="WFGraph (strict)"(error in=w141, "XScale.Offset"=w139) -> (error out=w140:errorcluster)  [unwired: 1 in, 1 out]
      }
      frame "TimeShift" {
        n90 = Unbundle("Index#") -> (w183:dbl, w181:dbl)
        n91 = Decrement(x=w181) -> (x-1=w178:dbl)
        n92 = To Unsigned Long Integer(number=w183) -> (unsigned 32bit integer=w188:u32)
        n93 = To Unsigned Long Integer(number=w178) -> (unsigned 32bit integer=w182:u32)
        n94 = Build Array(w188) -> (w184:u32[])
        n95 = Build Array(w182) -> (w180:u32[])
        n96 = control-ref of="TimeString (Low)"() -> (w185:refnum<vi>)
        n97 = property class="Arr (strict)"(reference=w185, error in=w187, "Index Values"=w184) -> (error out=w186:errorcluster)  [unwired: 1 out]
        n98 = control-ref of="TimeString (High)"() -> (w179:refnum<vi>)
        n99 = property class="Arr (strict)"(reference=w179, "Index Values"=w180) -> ()  [unwired: 1 in, 2 out]
      }
      frame "Exit" {
      }
    }
    n100 = call "Log_Errors_20190313.vi"("LoopName"="Main", "error in"=w48) -> ("error out"=w47:errorcluster)  [unwired: 9 in]
  }
  n101 = call "TreeItemsFromGroupName.vi"() -> ()  [unwired: 9 in, 3 out]
